vi "Flow-Meter-Testing.vi"() -> ()   [LabVIEW 2019]
uses:
  <vilib>/MakerHub/LINX/Public/Peripherals/Analog/Analog Read 1 Chan.vi
  <vilib>/MakerHub/LINX/Public/Peripherals/Analog/Analog Read N Chans.vi
  <vilib>/MakerHub/LINX/Private/Local IO/LinxAnalogRead.vi
  <vilib>/MakerHub/LINX/Public/Utilities/Check Channel.vi
  <vilib>/MakerHub/LINX/Public/Utilities/Open Serial.vi
  <vilib>/MakerHub/LINX/Private/Utilties/Generate Error.vi
  <vilib>/MakerHub/LINX/LMH-LINX.lvlib
panel:
  out "Flow-4":dbl
  in  "Cal-4":dbl
  out "Flow-3":dbl
  in  "Cal-3":dbl
  out "Flow-1":dbl
  in  "Cal-1":dbl
  out "Flow-2":dbl
  in  "Cal-2":dbl
  out "Flow-0":dbl
  in  "Cal-0":dbl
  out "VCH-4":dbl
  out "VCH-3":dbl
  out "VCH-1":dbl
  out "VCH-2":dbl
  out "VCH-0":dbl
  in  "Stop Measurement":bool
  in  "Measurement Rate (ms)":u32
  # "VOLTAGE (V)"
  # "CALIBRATION CONSTANT"
  # "FLOW READING"
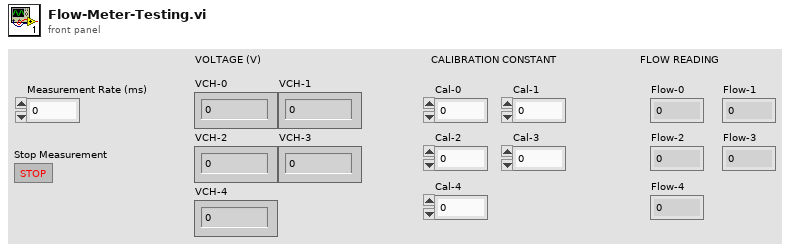
[diagram p1: front panel]
types:
  T1 = typedef "LMH-LINX.lvlib/LINX Ref.ctl" = cluster{"IO":T2, "Interface":T3, "LINX Device Config":T4}
  T2 = typedef "LMH-LINX.lvlib/Platform.ctl" = enum16{"Remote", "Local"}
  T3 = typedef "LMH-LINX.lvlib/Interface.ctl" = enum16{"Serial", "TCP"}
  T4 = typedef "LMH-LINX.lvlib/Device.lvlib/LINX Device Config.ctl" = cluster{"Interface":T3, "COM Port":refnum<visa-resource-name>, "TCP Configuration":T5, "Device Family":u8, "Device ID":u8, "Device Name":string, "TCP Ref":refnum<k5>, "Channels":T6}
  T5 = typedef "LMH-LINX.lvlib/Device.lvlib/TCP Config.ctl" = cluster{"IP Address":string, "Port":u16}
  T6 = typedef "LMH-LINX.lvlib/Channels.ctl" = cluster{"DI":u8[], "DO":u8[], "AI":u8[], "AO":u8[], "PWM":u8[], "QE":u8[], "UART":u8[], "I2C 2":u8[], "SPI":u8[], "CAN":u8[], "Servo":u8[], "AI Ref (V)":dbl, "AI Resolution (Bits)":u8, "AO Ref (V)":dbl, "AO Resolution (Bits)":u8}
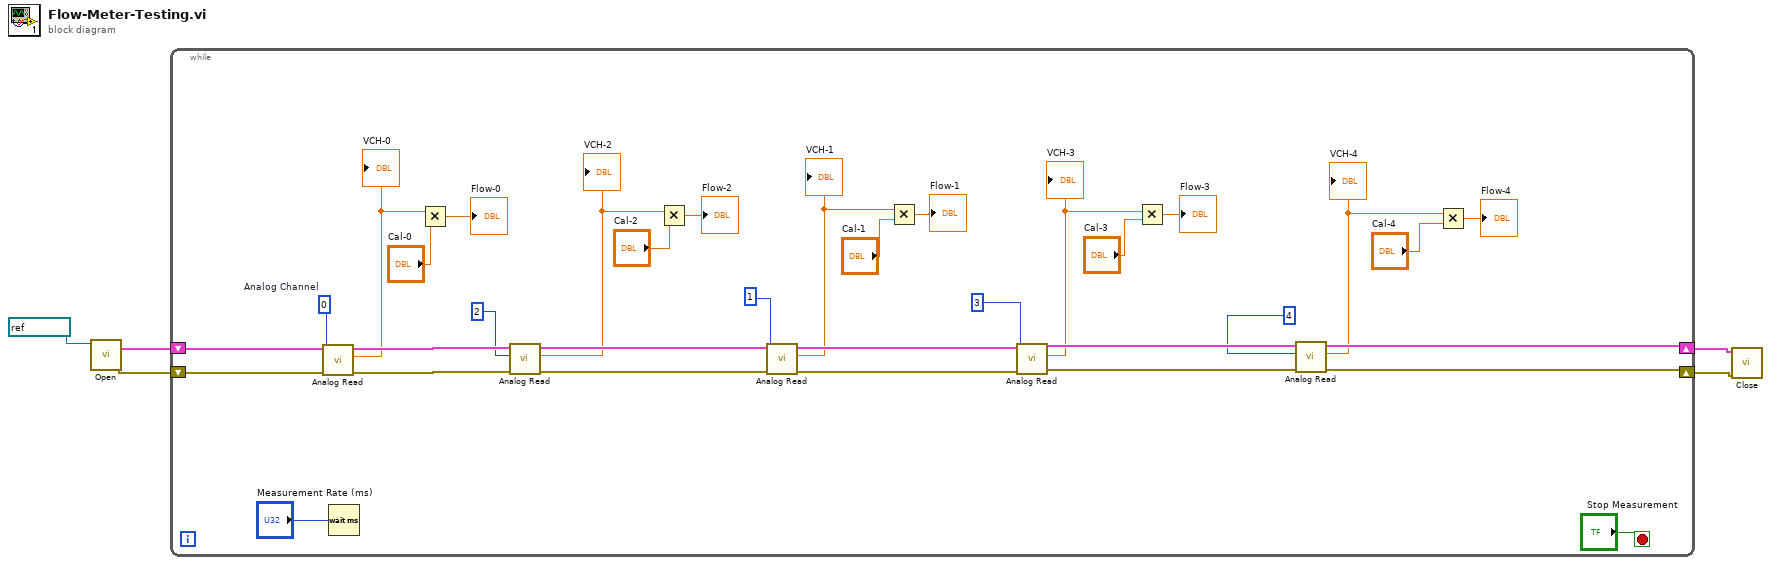
[diagram p0: block diagram]
diagram:
  n1 = call-poly <vilib>:"Open.vi"("Serial Port"=refnum<visa-resource-name> "COM3") -> ("Error Out"=w4:errorcluster, "LINX Resource"=w3:T1)  [unwired: 8 in, 1 out]
  n2 = while {
    shift-right: [w30] -> w1
    shift-left: w4 -> [w38]
    shift-right: [w31] -> w2
    shift-left: w3 -> [w37]
    stop <- "Stop Measurement" stop-if-true
    w39 = u8 0  # Analog Channel
    n3 = call-poly <vilib>:"Analog Read.vi"("Error In"=w38, "Analog Channel"=w39, "LINX Resource"=w37) -> ("Error Out"=w35:errorcluster, "Voltage"=w20:dbl, "LINX Resource"=w36:T1)  [unwired: 5 in, 1 out]
    "VCH-0" <- w20
    n4 = Wait (ms)(milliseconds to wait="Measurement Rate (ms)") -> ()  [unwired: 1 out]
    n5 = Multiply(x=w20, y="Cal-0") -> (x*y=→"Flow-0":dbl)
    n6 = call-poly <vilib>:"Analog Read.vi"("Error In"=w35, "Analog Channel"=u8 2, "LINX Resource"=w36) -> ("Error Out"=w23:errorcluster, "Voltage"=w17:dbl, "LINX Resource"=w25:T1)  [unwired: 5 in, 1 out]
    "VCH-2" <- w17
    n7 = Multiply(x=w17, y="Cal-2") -> (x*y=→"Flow-2":dbl)
    n8 = call-poly <vilib>:"Analog Read.vi"("Error In"=w23, "Analog Channel"=u8 1, "LINX Resource"=w25) -> ("Error Out"=w22:errorcluster, "Voltage"=w14:dbl, "LINX Resource"=w24:T1)  [unwired: 5 in, 1 out]
    "VCH-1" <- w14
    n9 = Multiply(x=w14, y="Cal-1") -> (x*y=→"Flow-1":dbl)
    n10 = call-poly <vilib>:"Analog Read.vi"("Error In"=w22, "Analog Channel"=u8 3, "LINX Resource"=w24) -> ("Error Out"=w33:errorcluster, "Voltage"=w11:dbl, "LINX Resource"=w34:T1)  [unwired: 5 in, 1 out]
    "VCH-3" <- w11
    n11 = Multiply(x=w11, y="Cal-3") -> (x*y=→"Flow-3":dbl)
    n12 = call-poly <vilib>:"Analog Read.vi"("Error In"=w33, "Analog Channel"=u8 4, "LINX Resource"=w34) -> ("Error Out"=w30:errorcluster, "Voltage"=w8:dbl, "LINX Resource"=w31:T1)  [unwired: 5 in, 1 out]
    "VCH-4" <- w8
    n13 = Multiply(x=w8, y="Cal-4") -> (x*y=→"Flow-4":dbl)
  }
  n14 = call <vilib>:"Close.vi"("Error In"=w1, "LINX Resource"=w2) -> ()  [unwired: 9 in, 1 out]
